vi "Get GUI Enqueuer.vi"(11 "Series Actor in":refnum<class "Series Actor.lvclass">) -> (2 "Actor Framework:Message Enqueuer":refnum<class "Message Enqueuer.lvclass">, 3 "Series Actor out":refnum<class "Series Actor.lvclass">)   [LabVIEW 2024, in "Series Actor.lvlib" / "Series Actor.lvclass"]
uses:
  Series Actor.lvclass
  Series Actor.lvclass/Series Actor.ctl
  <vilib>/ActorFramework/Message Enqueuer/Message Enqueuer.lvclass
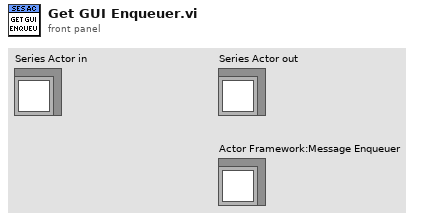
[diagram p1: front panel]
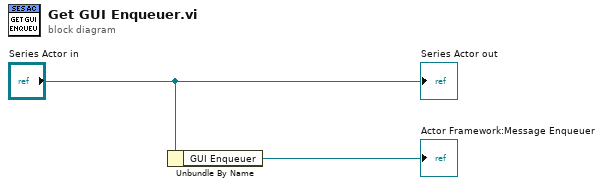
[diagram p0: block diagram]
diagram:
  n1 = Unbundle By Name("Series Actor in") -> ("GUI Enqueuer"=→"Actor Framework:Message Enqueuer":refnum<class "Message Enqueuer.lvclass">)
  "Series Actor out" <- "Series Actor in"
